vi "create_connection.vi"(0 "device_index (def=0)":i32, 11 "error in (no error)":errorcluster, 12 "clear_buffer? (T)":bool=TRUE) -> (4 "reference":i32, 15 "error out":errorcluster)   [LabVIEW 2020, in "classes.lvlib" / "_Controller.lvclass"]
doc: "Opens a reference to the specified device (takes as input device Index and outputs a device Reference). \n\nImplementss the USB Communication API function \"fnPerformaxCaomOpen\".\n\nNOTE: The \"index\" is determined by choosing the item from a list of queried items using the \"get_device_list.vi\" VI. Further note a USB Clear Buffer command is (by default) issued immediately after a connection is established in the event a previous session was not properly terminated. This feature is NOT supported in all versions of the API - therefore it may be bypassed by assigning a FALSE to the \"clear_buffer\" input.\n\nProduced By:\n\n<B>Kod Integrations, LLC</B>\n4835 Marianne Drive\nMount Airy, MD 21771\nhttp://www.kodintegrations.com\nemail: info@kodintegrations.com\nphone: (240) 687-1288"
uses:
  classes/Controller/_Controller.lvclass
  common/controls/error_actions.ctl
  PerformaxCom.dll
  libraries/common.lvlib
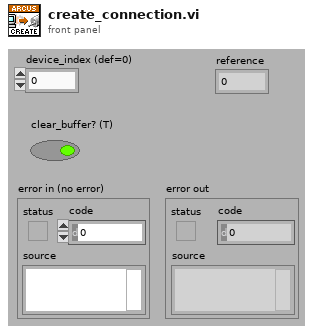
[diagram p1: front panel]
types:
  T1 = typedef "common.lvlib/error_actions.ctl" = enum16{"clearBuff", "closeRef", "nodeErr", "noDeviceInfo", "noDevices", "openRef", "sendReceive", "setTimeouts", "unknown"}
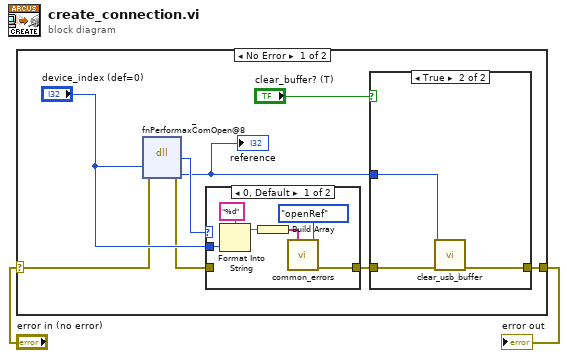
[diagram p0: block diagram]
diagram:
  n1 = case shown="No Error" "error in (no error)" {
    selector: "error in (no error)" -> [w4 w22]
    tunnel: [w6 w22] -> w1
    frame No Error {
      n2 = dll-call lib="PerformaxCom.dll" fn="_fnPerformaxComOpen@8"(error in=w4, "deviceIndex"="device_index (def=0)") -> (error out=w3:errorcluster, "success"=w10:i32, "reference"=w5:i32)  [unwired: 4 in, 1 out]
      "reference" <- w5
      n3 = case shown="0, Default" w10 {
        tunnel: [w19 w21] -> w7
        tunnel: w3 -> [_ w21]
        tunnel: "device_index (def=0)" -> [w18 _]
        frame 0, Default {
          n4 = Format Into String(format string="%d", w18) -> (resulting string=w16:string)  [unwired: 2 in, 1 out]
          n5 = Build Array(w16) -> (w15:string[])
          n6 = call "common_errors.vi"("common_errors"=error_actions."openRef" ("errors"), "supp_text"=w15) -> ("error out"=w19:errorcluster)  [unwired: 13 in]
        }
        frame 1 {
        }
      }
      n7 = case shown="True" "clear_buffer? (T)" {
        tunnel: w7 -> [w11 w14]
        tunnel: [w11 w13] -> w6
        tunnel: w5 -> [_ w12]
        frame False {
        }
        frame True {
          n8 = call "clear_usb_buffer.vi"("reference (in)"=w12, "error in (no error)"=w14) -> ("error out"=w13:errorcluster)  [unwired: 16 in, 1 out]
        }
      }
    }
    frame Error {
    }
  }
  "error out" <- w1
